vi "viktory.vi"() -> ()   [LabVIEW 2014]
uses:
  <vilib>/Platform/TimedLoop/XDataNode/timing_clust.ctl
  <vilib>/Platform/TimedLoop/XDataNode/nitl_modes.ctl
  <vilib>/Platform/TimedLoop/XDataNode/wakeup.ctl
  <vilib>/DAQmx/create/channels.llb/DAQmx Create Channel (AI-Voltage-Basic).vi
  <vilib>/DAQmx/configure/timing.llb/DAQmx Timing (Sample Clock).vi
  <vilib>/DAQmx/read.llb/DAQmx Read (Analog 2D DBL NChan NSamp).vi
  <vilib>/platform/TimedLoop/XDataNode/XDataNode.xnode
  <vilib>/Platform/TimedLoop/XDataNode/XDNodeRunTimeDep.lvlib
panel:
  out "Waveform Graph 3":dynamicdata(graph)
  out "Waveform Graph 2":dynamicdata(graph)
  out "Waveform Graph":dynamicdata(graph)
  out "angle":dbl
  out "Waveform Chart 6":i32(graph)
  out "Waveform Chart 5":i32(graph)
  out "Waveform Chart":dbl(graph)
  out "Waveform Chart 4":i32(graph)
  in  "physical channels":tag
  in  "stop":bool
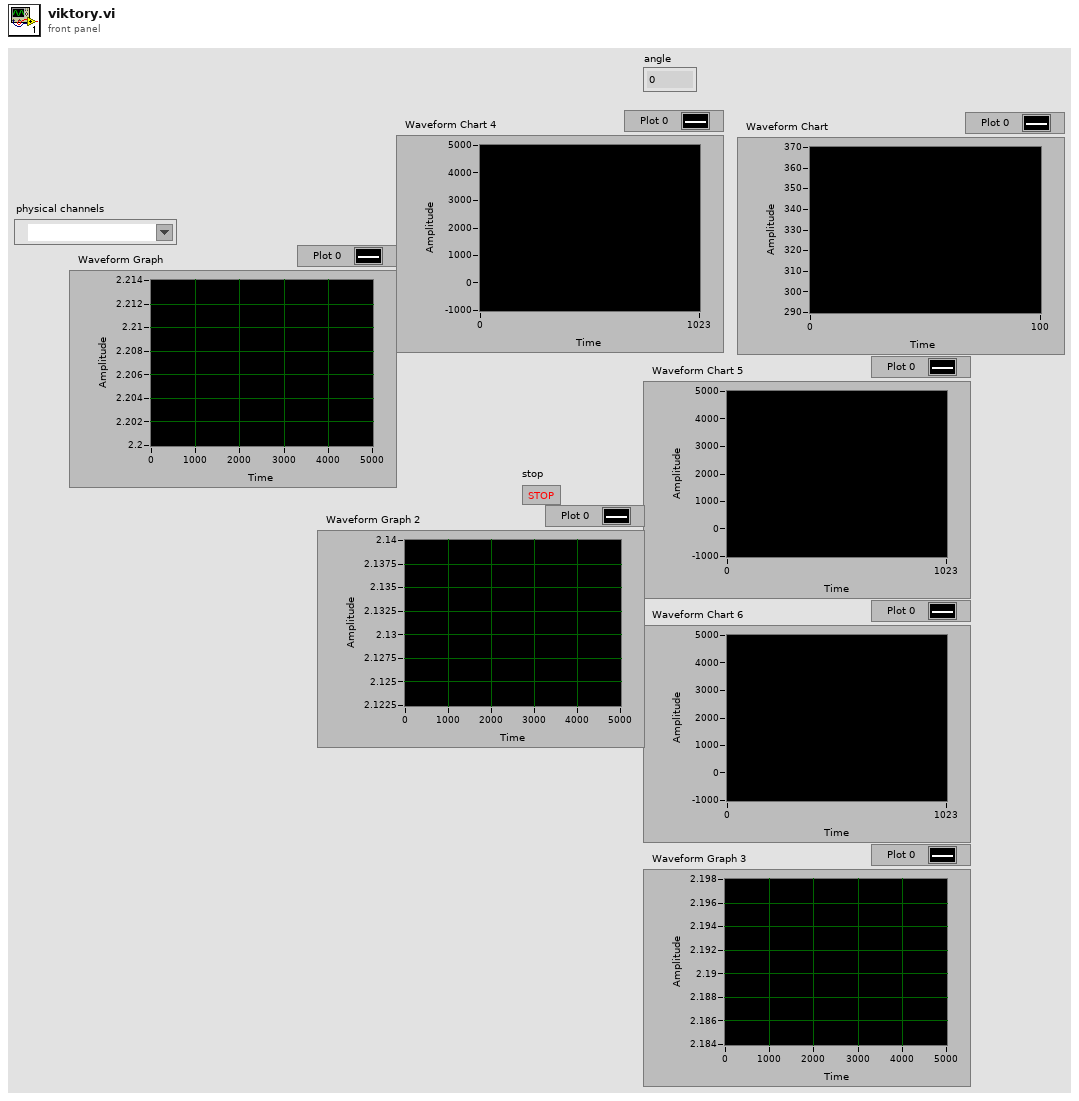
[diagram p1: front panel]
types:
  T1 = typedef "XDNodeRunTimeDep.lvlib/timing_clust.ctl" = cluster{"Expected End [f-1]":u64, "Actual End [f-1]":u64, "Finished Late? [f-1]":bool, "Expected End [i-1]":u64, "Actual End [i-1]":u64, "Finished Late? [i-1]":bool, "Expected Start [i]":u64, "Actual Start [i]":u64, "Expected Start [f]":u64, "Actual Start [f]":u64, "Source Name":string, "Structure Name":string, "Period":i64, "Deadline":i64, "Offset":i64, "Start":i64, "Priority":i32, "Timeout":i32, "Mode":T2, "Wakeup Reason":T3, "Error":errorcluster, "Source Type":string, "Secondary Source Type":string, "Global End Time":u64, "Global Start Time":u64, "Frame Duration":u64, "Iteration Duration":u64, "Assigned CPU":i32, "I/O Scan Engine Mode":u32}
  T2 = typedef "XDNodeRunTimeDep.lvlib/nitl_modes.ctl" = enum32{"No Change", "Process missed periods, maintain original phase", "Discard missed periods, maintain original phase", "Process missed periods, ignore original phase", "Discard missed periods, ignore original phase"}
  T3 = typedef "XDNodeRunTimeDep.lvlib/wakeup.ctl" = enum32{"Normal", "Aborted", "Asynchronous wakeup", "Timing source error", "Timed loop error", "Timeout"}
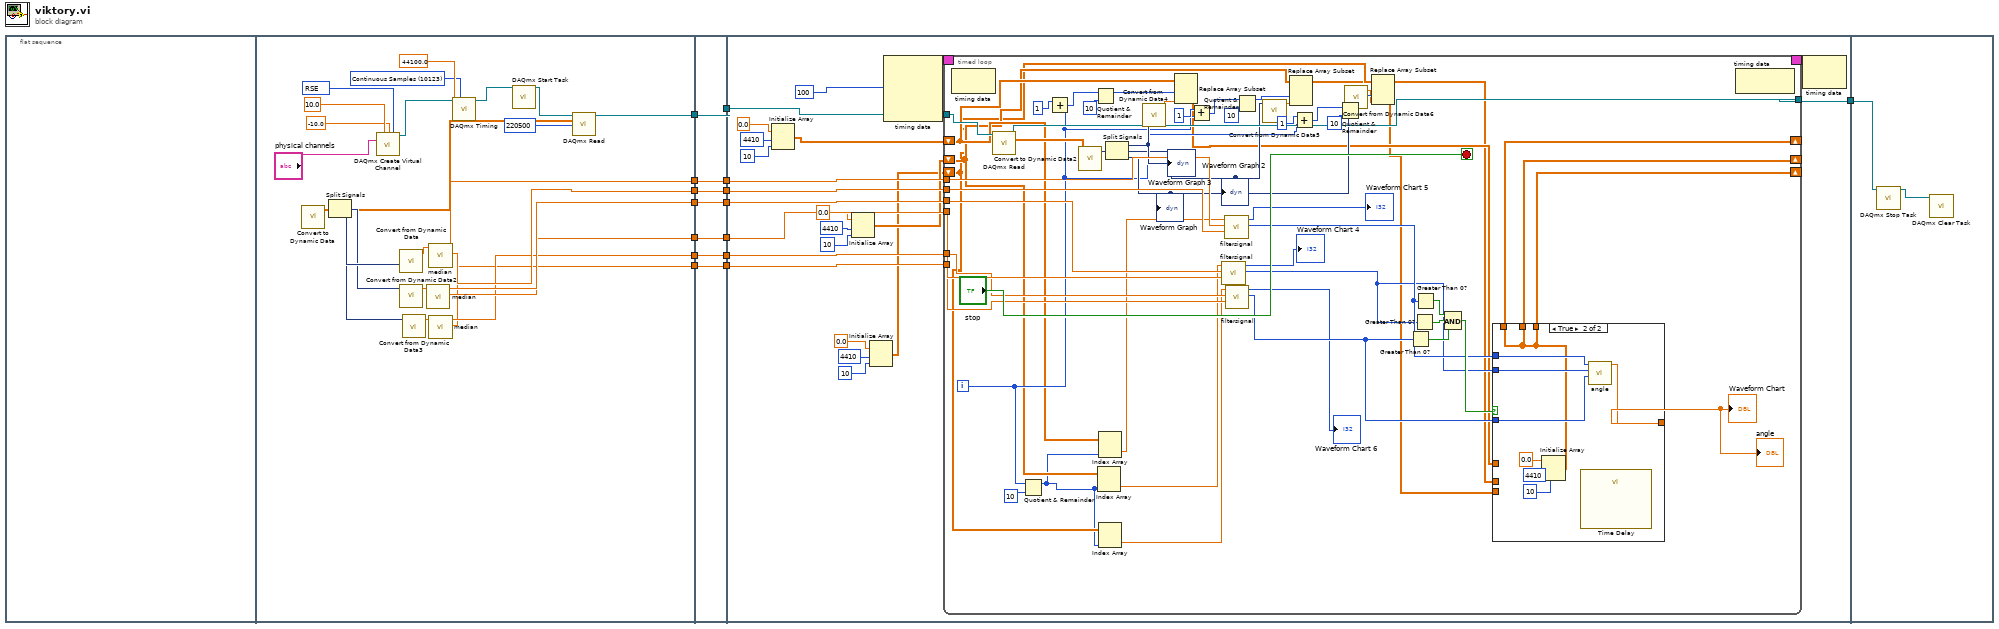
[diagram p0: block diagram]
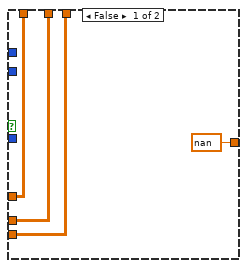
[diagram p2: hidden frame]
diagram:
  n1 = flat-sequence {
    tunnel: [w40] -> w15
    tunnel: [w33] -> w13
    tunnel: [w32] -> w11
    tunnel: [w31] -> w9
    tunnel: [w30] -> w7
    tunnel: [w29] -> w5
    tunnel: [w19] -> w3
    tunnel: w15 -> [w47]
    tunnel: [w47] -> w14
    tunnel: w13 -> [w46]
    tunnel: [w46] -> w12
    tunnel: w11 -> [w45]
    tunnel: [w45] -> w10
    tunnel: w9 -> [w44]
    tunnel: [w44] -> w8
    tunnel: w7 -> [w43]
    tunnel: [w43] -> w6
    tunnel: w5 -> [w42]
    tunnel: [w42] -> w4
    tunnel: w3 -> [w41]
    tunnel: [w41] -> w2
    tunnel: w14 -> [w70]
    tunnel: w12 -> [w69]
    tunnel: w10 -> [w68]
    tunnel: w8 -> [w67]
    tunnel: w6 -> [w66]
    tunnel: w4 -> [w65]
    tunnel: w2 -> [w63]
    tunnel: [w64] -> w1
    tunnel: w1 -> [w145]
    frame #0 {
    }
    frame #1 {
      w17 = 10123 items=["Finite Samples"=10178, "Continuous Samples"=10123, "Hardware Timed Single Point"=12522] ("sample mode")
      w27 = 10083 items=["default"=-1, "RSE"=10083, "NRSE"=10078, "Differential"=10106, "Pseudodifferential"=12529] ("input terminal configuration")
      n2 = call-poly <vilib>:"DAQmx Create Virtual Channel.vi"("maximum value"=10.0, "minimum value"=-10.0, "input terminal configuration"=w27, "physical channels"="physical channels") -> ("task out"=w24:refnum<k21>)  [unwired: 10 in, 1 out]
      n3 = call-poly <vilib>:"DAQmx Timing.vi"("task/channels in"=w24, "sample mode"=w17, "rate"=44100.0) -> ("task out"=w23:refnum<k21>)  [unwired: 11 in, 1 out]
      n4 = call <vilib>:"DAQmx Start Task.vi"("task/channels in"=w23) -> ("task out"=w22:refnum<k21>)  [unwired: 13 in, 1 out]
      n5 = call-poly <vilib>:"DAQmx Read.vi"("task/channels in"=w22, "number of samples per channel"=220500) -> ("task out"=w19:refnum<k21>, "data"=w21:dbl[][])  [unwired: 11 in, 1 out]
      n6 = call "Convert to Dynamic Data"("2D Array"=w21) -> ("Dynamic Data Type"=w20:dynamicdata)  [unwired: 3 in]
      n7 = Split Signals(w20) -> (w39:dynamicdata, w37:dynamicdata, w35:dynamicdata)  [unwired: 3 in]
      n8 = call "Convert from Dynamic Data"("Dynamic Data Type"=w39) -> ("Array"=w38:dbl[])  [unwired: 3 in]
      n9 = call "Convert from Dynamic Data2"("Dynamic Data Type"=w37) -> ("Array"=w36:dbl[])  [unwired: 3 in]
      n10 = call "Convert from Dynamic Data3"("Dynamic Data Type"=w35) -> ("Array"=w34:dbl[])  [unwired: 3 in]
      n11 = call "median.vi"("Array"=w36) -> ("s"=w31:dbl, "m"=w32:dbl)  [unwired: 9 in]
      n12 = call "median.vi"("Array"=w38) -> ("s"=w33:dbl, "m"=w40:dbl)  [unwired: 9 in]
      n13 = call "median.vi"("Array"=w34) -> ("s"=w29:dbl, "m"=w30:dbl)  [unwired: 9 in]
    }
    frame #2 {
    }
    frame #3 {
      n14 = Initialize Array(0.0 ("element"), 4410 ("dimension size"), 10 ("dimension size")) -> (w56:dbl[][])
      n15 = Initialize Array(0.0 ("element"), 4410 ("dimension size"), 10 ("dimension size")) -> (w52:dbl[][])
      n16 = Initialize Array(0.0 ("element"), 4410 ("dimension size"), 10 ("dimension size")) -> (w48:dbl[][])
      n17 = node-c288(i64 100 ("Period")) -> (w62:T1)  [unwired: 3 in]
      n18 = timed-loop {
        tunnel: w70 -> [w124]
        tunnel: w69 -> [w123]
        tunnel: w68 -> [w122]
        tunnel: w67 -> [w121]
        tunnel: w66 -> [w120]
        tunnel: w65 -> [w119]
        tunnel: [w118] -> w64
        tunnel: w63 -> [w117]
        timing: w62 -> [_]
        timing-out: [_] -> w61
        shift-right: [w74] -> _
        shift-left: w56 -> [w83]
        shift-right: [w73] -> _
        shift-left: w52 -> [w81]
        shift-right: [w72] -> _
        shift-left: w48 -> [w79]
        i -> [w84]
        stop <- "stop" stop-if-true
        n19 = node-c288() -> ()  [unwired: 1 in, 1 out]
        n20 = call-poly <vilib>:"DAQmx Read.vi"("task/channels in"=w117) -> ("task out"=w118:refnum<k21>, "data"=w116:dbl[][])  [unwired: 12 in, 1 out]
        n21 = Quotient & Remainder(x=w84, y=10) -> (x-y*floor(x/y)=w78:i32)  [unwired: 1 out]
        n22 = Add(x=1, y=w84) -> (x+y=w111:i32)
        n23 = call "Convert to Dynamic Data2"("2D Array"=w116) -> ("Dynamic Data Type"=w115:dynamicdata)  [unwired: 3 in]
        n24 = Quotient & Remainder(x=w111, y=10) -> (x-y*floor(x/y)=w113:i32)  [unwired: 1 out]
        n25 = Index Array(array=w81, index (col)=w78) -> (element=w80:dbl[])  [unwired: 1 in]
        n26 = Index Array(array=w83, index (col)=w78) -> (element=w82:dbl[])  [unwired: 1 in]
        n27 = Index Array(array=w79, index (col)=w78) -> (element=w77:dbl[])  [unwired: 1 in]
        n28 = Split Signals(w115) -> (w110:dynamicdata, w89:dynamicdata, w87:dynamicdata)  [unwired: 3 in]
        "Waveform Graph" <- w87
        "Waveform Graph 2" <- w89
        "Waveform Graph 3" <- w110
        n29 = call "Convert from Dynamic Data4"("Dynamic Data Type"=w110) -> ("Array"=w109:dbl[])  [unwired: 3 in]
        n30 = Replace Array Subset(array=w83, new element=w109, index (col)=w113) -> (w76:dbl[][])  [unwired: 1 in]
        n31 = Add(x=1, y=w84) -> (x+y=w106:i32)
        n32 = call "filtersignal.vi"("Array"=w80, "m"=w122, "3s"=w121) -> ("Waveform Chart 2"=→"Waveform Chart 4":i32, "Numeric"=w94:i32)  [unwired: 5 in]
        n33 = call "filtersignal.vi"("Array"=w82, "m"=w124, "3s"=w123) -> ("Waveform Chart 2"=→"Waveform Chart 5":i32, "Numeric"=w95:i32)  [unwired: 5 in]
        n34 = call "filtersignal.vi"("Array"=w77, "m"=w120, "3s"=w119) -> ("Waveform Chart 2"=→"Waveform Chart 6":i32, "Numeric"=w93:i32)  [unwired: 5 in]
        n35 = Quotient & Remainder(x=w106, y=10) -> (x-y*floor(x/y)=w105:i32)  [unwired: 1 out]
        n36 = call "Convert from Dynamic Data5"("Dynamic Data Type"=w89) -> ("Array"=w88:dbl[])  [unwired: 3 in]
        n37 = Replace Array Subset(array=w81, new element=w88, index (col)=w105) -> (w71:dbl[][])  [unwired: 1 in]
        n38 = Add(x=1, y=w84) -> (x+y=w102:i32)
        n39 = Quotient & Remainder(x=w102, y=10) -> (x-y*floor(x/y)=w101:i32)  [unwired: 1 out]
        n40 = call "Convert from Dynamic Data6"("Dynamic Data Type"=w87) -> ("Array"=w86:dbl[])  [unwired: 3 in]
        n41 = Replace Array Subset(array=w79, new element=w86, index (col)=w101) -> (w75:dbl[][])  [unwired: 1 in]
        n42 = Greater Than 0?(x=w93) -> (x > 0?=w96:bool)
        n43 = Greater Than 0?(x=w94) -> (x > 0?=w97:bool)
        n44 = Greater Than 0?(x=w95) -> (x > 0?=w98:bool)
        n45 = Compound Arithmetic op=AND(w98, w97, w96) -> (w99:bool)
        n46 = case shown="True" w99 {
          tunnel: [nan ("angle") w139] -> w92
          tunnel: w95 -> [_ w138]
          tunnel: w94 -> [_ w137]
          tunnel: w93 -> [_ w136]
          tunnel: w76 -> [w130 _]
          tunnel: w71 -> [w129 _]
          tunnel: w75 -> [w128 _]
          tunnel: [w130 w132] -> w74
          tunnel: [w129 w132] -> w73
          tunnel: [w128 w132] -> w72
          frame False {
          }
          frame True {
            n47 = Initialize Array(0.0 ("element"), 4410 ("dimension size"), 10 ("dimension size")) -> (w132:dbl[][])
            n48 = call "Time Delay"() -> ()  [unwired: 11 in, 1 out]
            n49 = call "angle.vi"("mic3"=w136, "mic2"=w137, "mic1"=w138) -> ("angle"=w139:dbl)  [unwired: 8 in]
          }
        }
        "Waveform Chart" <- w92
        "angle" <- w92
        n50 = node-c288() -> ()  [unwired: 1 in, 1 out]
      }
      n51 = node-c288(w61) -> ()  [unwired: 1 out]
    }
    frame #4 {
      n52 = call <vilib>:"DAQmx Stop Task.vi"("task/channels in"=w145) -> ("task out"=w144:refnum<k21>)  [unwired: 13 in, 1 out]
      n53 = call <vilib>:"DAQmx Clear Task.vi"("task in"=w144) -> ()  [unwired: 14 in, 1 out]
    }
  }
